vi "VI Tree.vi"   [LabVIEW 2017, in "Tektronix TDS 200 1000 2000 Series.lvlib"]
doc: "This is the instrument driver for Tektronix TDS 200, 1000, and 2000 Series oscilliscopes. The VI Tree displays all the user-callable VIs of the instrument driver in an organized table."
uses:
  Tektronix TDS 200 1000 2000 Series.lvlib
  Configure/Configure Trigger (Edge).vi
  Data/Read (Single Waveform).vi
panel:
  # "(C) 2009-2015 National Instruments.  ALL RIGHTS RESERVED."
  # "SEE DIAGRAM\nFOR VI TREE."
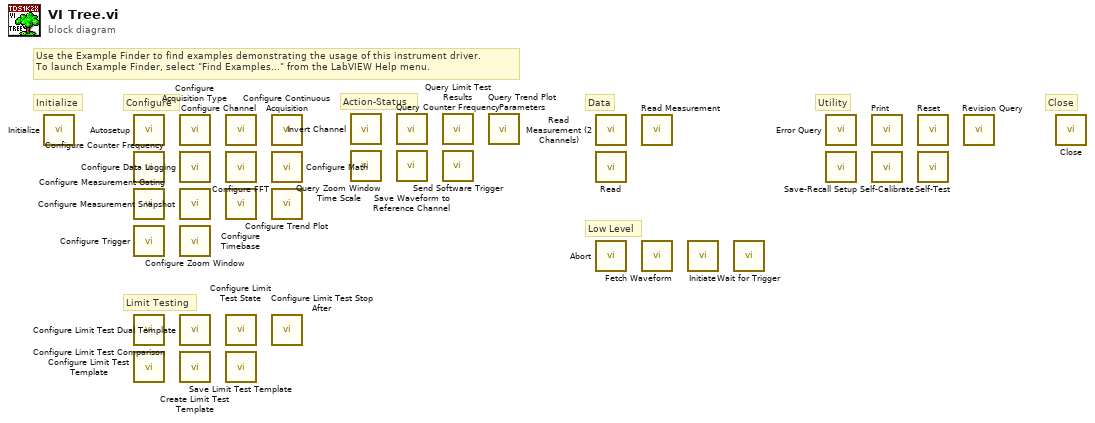
[diagram p0: block diagram]
diagram:
  # "Close"
  # "Utility"
  # "Low Level"
  # "Data"
  # "Limit Testing"
  # "Configure"
  # "Action-Status"
  # "Initialize"
  # "Use the Example Finder to find examples demonstrating the usage of this instrument driver.\nTo launch Example Finder, select \"Find Examples...\" from the LabVIEW Help menu."
  n1 = call "Initialize.vi"() -> ()  [unwired: 10 in, 2 out]
  n2 = call "Autosetup.vi"() -> ()  [unwired: 10 in, 2 out]
  n3 = call "Configure Counter Frequency.vi"() -> ()  [unwired: 10 in, 2 out]
  n4 = call "Configure Measurement Gating.vi"() -> ()  [unwired: 10 in, 2 out]
  n5 = call-poly "Configure Trigger.vi"() -> ()  [unwired: 14 in, 2 out]
  n6 = call "Configure Limit Test Comparison.vi"() -> ()  [unwired: 10 in, 2 out]
  n7 = call "Configure Limit Test Template.vi"() -> ()  [unwired: 10 in, 2 out]
  n8 = call "Configure Acquisition Type.vi"() -> ()  [unwired: 10 in, 2 out]
  n9 = call "Configure Data Logging.vi"() -> ()  [unwired: 10 in, 2 out]
  n10 = call "Configure Measurement Snapshot.vi"() -> ()  [unwired: 10 in, 2 out]
  n11 = call "Configure Zoom Window.vi"() -> ()  [unwired: 10 in, 2 out]
  n12 = call "Configure Limit Test Dual Template.vi"() -> ()  [unwired: 10 in, 2 out]
  n13 = call "Create Limit Test Template.vi"() -> ()  [unwired: 10 in, 2 out]
  n14 = call "Configure Channel.vi"() -> ()  [unwired: 14 in, 2 out]
  n15 = call "Configure FFT.vi"() -> ()  [unwired: 10 in, 2 out]
  n16 = call "Configure Timebase.vi"() -> ()  [unwired: 10 in, 2 out]
  n17 = call "Configure Limit Test State.vi"() -> ()  [unwired: 10 in, 2 out]
  n18 = call "Save Limit Test Template.vi"() -> ()  [unwired: 10 in, 2 out]
  n19 = call "Configure Continuous Acquisition.vi"() -> ()  [unwired: 10 in, 2 out]
  n20 = call "Configure Math.vi"() -> ()  [unwired: 10 in, 2 out]
  n21 = call "Configure Trend Plot.vi"() -> ()  [unwired: 10 in, 2 out]
  n22 = call "Configure Limit Test Stop After.vi"() -> ()  [unwired: 10 in, 2 out]
  n23 = call "Invert Channel.vi"() -> ()  [unwired: 10 in, 2 out]
  n24 = call "Query Zoom Window Time Scale.vi"() -> ()  [unwired: 9 in, 3 out]
  n25 = call "Query Counter Frequency.vi"() -> ()  [unwired: 9 in, 3 out]
  n26 = call "Save Waveform to Reference Channel.vi"() -> ()  [unwired: 10 in, 2 out]
  n27 = call "Query Limit Test Results.vi"() -> ()  [unwired: 7 in, 5 out]
  n28 = call "Send Software Trigger.vi"() -> ()  [unwired: 10 in, 2 out]
  n29 = call "Query Trend Plot Parameters.vi"() -> ()  [unwired: 6 in, 10 out]
  n30 = call "Read Measurement (2 Channels).vi"() -> ()  [unwired: 8 in, 4 out]
  n31 = call-poly "Read.vi"() -> ()  [unwired: 9 in, 3 out]
  n32 = call "Abort.vi"() -> ()  [unwired: 10 in, 2 out]
  n33 = call "Read Measurement.vi"() -> ()  [unwired: 8 in, 4 out]
  n34 = call "Fetch Waveform.vi"() -> ()  [unwired: 9 in, 3 out]
  n35 = call "Initiate.vi"() -> ()  [unwired: 10 in, 2 out]
  n36 = call "Wait for Trigger.vi"() -> ()  [unwired: 10 in, 2 out]
  n37 = call "Error Query.vi"() -> ()  [unwired: 8 in, 4 out]
  n38 = call "Save-Recall Setup.vi"() -> ()  [unwired: 10 in, 2 out]
  n39 = call "Print.vi"() -> ()  [unwired: 10 in, 2 out]
  n40 = call "Self-Calibrate.vi"() -> ()  [unwired: 9 in, 3 out]
  n41 = call "Reset.vi"() -> ()  [unwired: 10 in, 2 out]
  n42 = call "Self-Test.vi"() -> ()  [unwired: 8 in, 4 out]
  n43 = call "Revision Query.vi"() -> ()  [unwired: 8 in, 4 out]
  n44 = call "Close.vi"() -> ()  [unwired: 11 in, 1 out]
